vi "test_DevDIStatus.vi"() -> ()   [LabVIEW 2014]
panel:
  out "cluster":T1
  out "x-1":dbl
  in  "Boolean 3":bool
  in  "Boolean 2":bool
  in  "Boolean":bool
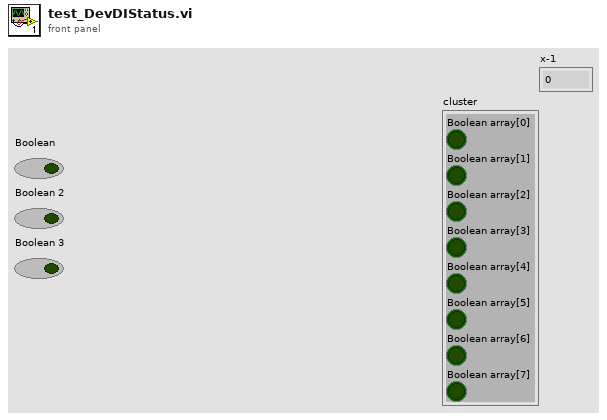
[diagram p1: front panel]
types:
  T1 = cluster{"Boolean array[0]":bool, "Boolean array[1]":bool, "Boolean array[2]":bool, "Boolean array[3]":bool, "Boolean array[4]":bool, "Boolean array[5]":bool, "Boolean array[6]":bool, "Boolean array[7]":bool}
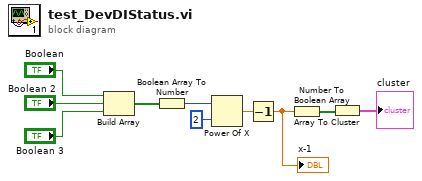
[diagram p0: block diagram]
diagram:
  n1 = Build Array("Boolean", "Boolean 2", "Boolean 3") -> (w7:bool[])
  n2 = Boolean Array To Number(Boolean array=w7) -> (number=w6:u32)
  n3 = Power Of X(1:u32 2 ("x"), 2:w6) -> (0:w4:dbl)
  n4 = Decrement(x=w4) -> (x-1=w3:dbl)
  "x-1" <- w3
  n5 = Number To Boolean Array(number=w3) -> (Boolean array=w2:bool[])
  n6 = Array To Cluster(array=w2) -> (cluster=→"cluster":T1)
